vi "Web Browser.vi"() -> ()   [LabVIEW 2024]
uses:
  WebView_class/WebView.lvclass
  <vilib>/sklein/WebView2/Libs/Microsoft.Web.WebView2.WinForms.dll
panel:
  in  "Stop":bool
  in  "Forward":bool
  in  "Backward":bool
  in  "Go":bool
  in  "URL":string="https://www.ni.com"
  in  "WebView2 Control in":refnum<k24>(container)
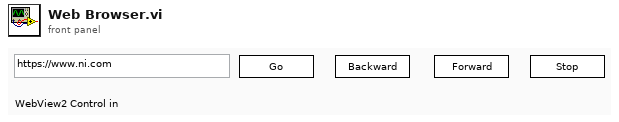
[diagram p1: front panel]
types:
  T1 = typedef "WebView.lvclass/Events--cluster.ctl" = cluster{"Navigation Complete Event":refnum<user-event>, "Source Changed Event":refnum<user-event>, "Document Title Changed Event":refnum<user-event>, "Status Bar Text Changed":refnum<user-event>, "Web Message Received":refnum<user-event>, "Window Close Requested":refnum<user-event>, "DOM Loaded":refnum<user-event>, "Navigation Started Event":refnum<user-event>}
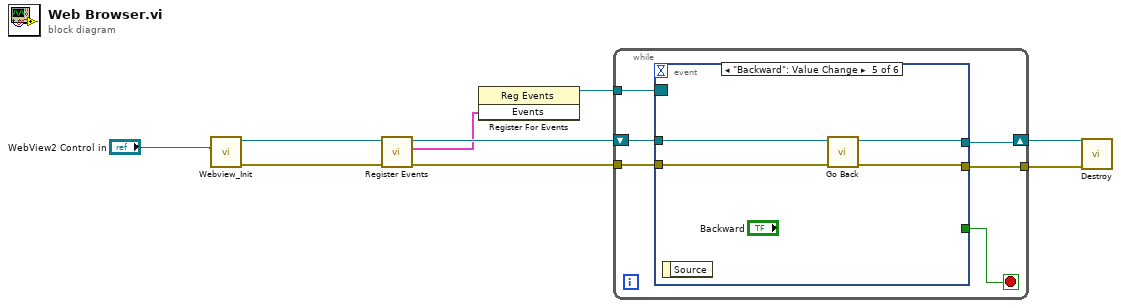
[diagram p0: block diagram]
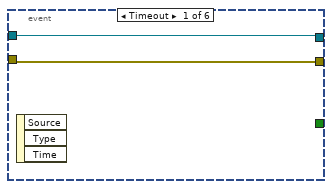
[diagram p2: hidden frame]
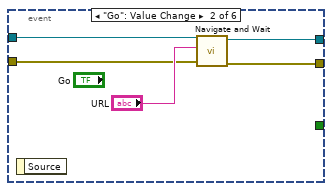
[diagram p3: hidden frame]
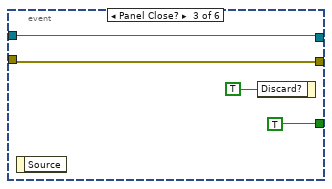
[diagram p4: hidden frame]
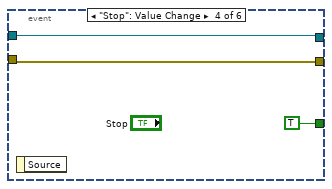
[diagram p5: hidden frame]
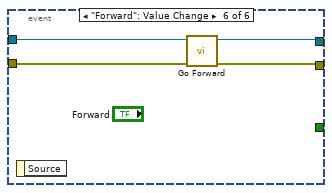
[diagram p6: hidden frame]
diagram:
  n1 = call "Webview_Init.vi"("WebView2 Control in"="WebView2 Control in") -> ("Error Out"=w5:errorcluster, "object out"=w6:refnum<class "WebView.lvclass">)  [unwired: 9 in]
  n2 = call-dynamic "Register Events.vi"("Error In"=w5, "object in"=w6) -> ("Error Out"=w4:errorcluster, "Events"=w2:T1, "object out"=w3:refnum<class "WebView.lvclass">)  [unwired: 7 in]
  n3 = register-events(w2) -> (reference out=w1:refnum<event-registration>)  [unwired: 2 in, 1 out]
  n4 = while {
    tunnel: w4 -> [w14]
    shift-right: [w13] -> w8
    shift-left: w3 -> [w15]
    tunnel: [w12] -> w7
    tunnel: w1 -> [w11]
    stop <- w10 stop-if-true
    n5 = event shown="[4] \"Backward\": Value Change" {
      selector: w11 -> [_ _ _ _ _ _]
      dyn-events: _ -> [_ _ _ _ _ _]
      timeout: _ -> [_ _ _ _ _ _]
      tunnel: w15 -> [w17 w21 w24 w29 w33 w37]
      tunnel: w14 -> [w16 w18 w23 w28 w32 w35]
      tunnel: [w17 w20 w24 w29 w31 w36] -> w13
      tunnel: [w16 w19 w23 w28 w30 w34] -> w12
      tunnel: [_ _ TRUE TRUE _ _] -> w10
      event Timeout {
        n6 = event-data() -> ()  [unwired: 1 in, 3 out]
      }
      event "Go": Value Change {
        n7 = event-data() -> ()  [unwired: 1 in, 1 out]
        n8 = call "Navigate and Wait.vi"("Error In"=w18, "Source"="URL", "object in"=w21) -> ("Error Out"=w19:errorcluster, "object out"=w20:refnum<class "WebView.lvclass">)  [unwired: 6 in, 1 out]
      }
      event Panel Close? {
        n9 = event-data() -> ()  [unwired: 1 in, 1 out]
        n10 = event-data("Discard?"=TRUE) -> ()  [unwired: 1 in, 1 out]
      }
      event "Stop": Value Change {
        n11 = event-data() -> ()  [unwired: 1 in, 1 out]
      }
      event "Backward": Value Change {
        n12 = event-data() -> ()  [unwired: 1 in, 1 out]
        n13 = call "Go Back.vi"("Error In"=w32, "object in"=w33) -> ("Error Out"=w30:errorcluster, "object out"=w31:refnum<class "WebView.lvclass">)  [unwired: 8 in]
      }
      event "Forward": Value Change {
        n14 = event-data() -> ()  [unwired: 1 in, 1 out]
        n15 = call "Go Forward.vi"("Error In"=w35, "object in"=w37) -> ("Error Out"=w34:errorcluster, "object out"=w36:refnum<class "WebView.lvclass">)  [unwired: 8 in]
      }
    }
  }
  n16 = call-dynamic "Destroy.vi"("Error In"=w7, "WebView"=w8) -> ()  [unwired: 9 in, 1 out]
